vi "Data write draft.vi"() -> ()   [LabVIEW 2012]
uses:
  <vilib>/Platform/TimedLoop/XDataNode/timing_clust.ctl
  <vilib>/Platform/TimedLoop/XDataNode/nitl_modes.ctl
  <vilib>/Platform/TimedLoop/XDataNode/wakeup.ctl
  Labview_Spring2014/EXO200-LabView Dec.8/LabView Dec.8/SubVi's/Connection Variable 1.vi
  <vilib>/addons/database/Connection.llb/Conn Execute.vi
  <vilib>/addons/database/Recordset.llb/Rec Destroy - Connection.vi
  <vilib>/Platform/TimedLoop/XDataNode/XDataNode.xnode
  <vilib>/addons/database/NI_Database_API.lvlib
  Labview_Spring2014/SQL project lib.lvlib
  <vilib>/Platform/TimedLoop/XDataNode/XDNodeRunTimeDep.lvlib
panel:
  out "Time":string
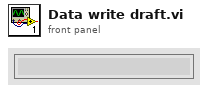
[diagram p1: front panel]
types:
  T1 = typedef "XDNodeRunTimeDep.lvlib/timing_clust.ctl" = cluster{"Expected End [f-1]":u64, "Actual End [f-1]":u64, "Finished Late? [f-1]":bool, "Expected End [i-1]":u64, "Actual End [i-1]":u64, "Finished Late? [i-1]":bool, "Expected Start [i]":u64, "Actual Start [i]":u64, "Expected Start [f]":u64, "Actual Start [f]":u64, "Source Name":string, "Structure Name":string, "Period":i64, "Deadline":i64, "Offset":i64, "Start":i64, "Priority":i32, "Timeout":i32, "Mode":T2, "Wakeup Reason":T3, "Error":errorcluster, "Source Type":string, "Secondary Source Type":string, "Global End Time":u64, "Global Start Time":u64, "Frame Duration":u64, "Iteration Duration":u64, "Assigned CPU":i32, "I/O Scan Engine Mode":u32}
  T2 = typedef "XDNodeRunTimeDep.lvlib/nitl_modes.ctl" = enum32{"No Change", "Process missed periods, maintain original phase", "Discard missed periods, maintain original phase", "Process missed periods, ignore original phase", "Discard missed periods, ignore original phase"}
  T3 = typedef "XDNodeRunTimeDep.lvlib/wakeup.ctl" = enum32{"Normal", "Aborted", "Asynchronous wakeup", "Timing source error", "Timed loop error", "Timeout"}
  T4 = typedef "NI_Database_API.lvlib/Conn ObjectReference.ctl" = refnum<k1>
  T5 = typedef "NI_Database_API.lvlib/Rec ObjectReference.ctl" = refnum<k1>
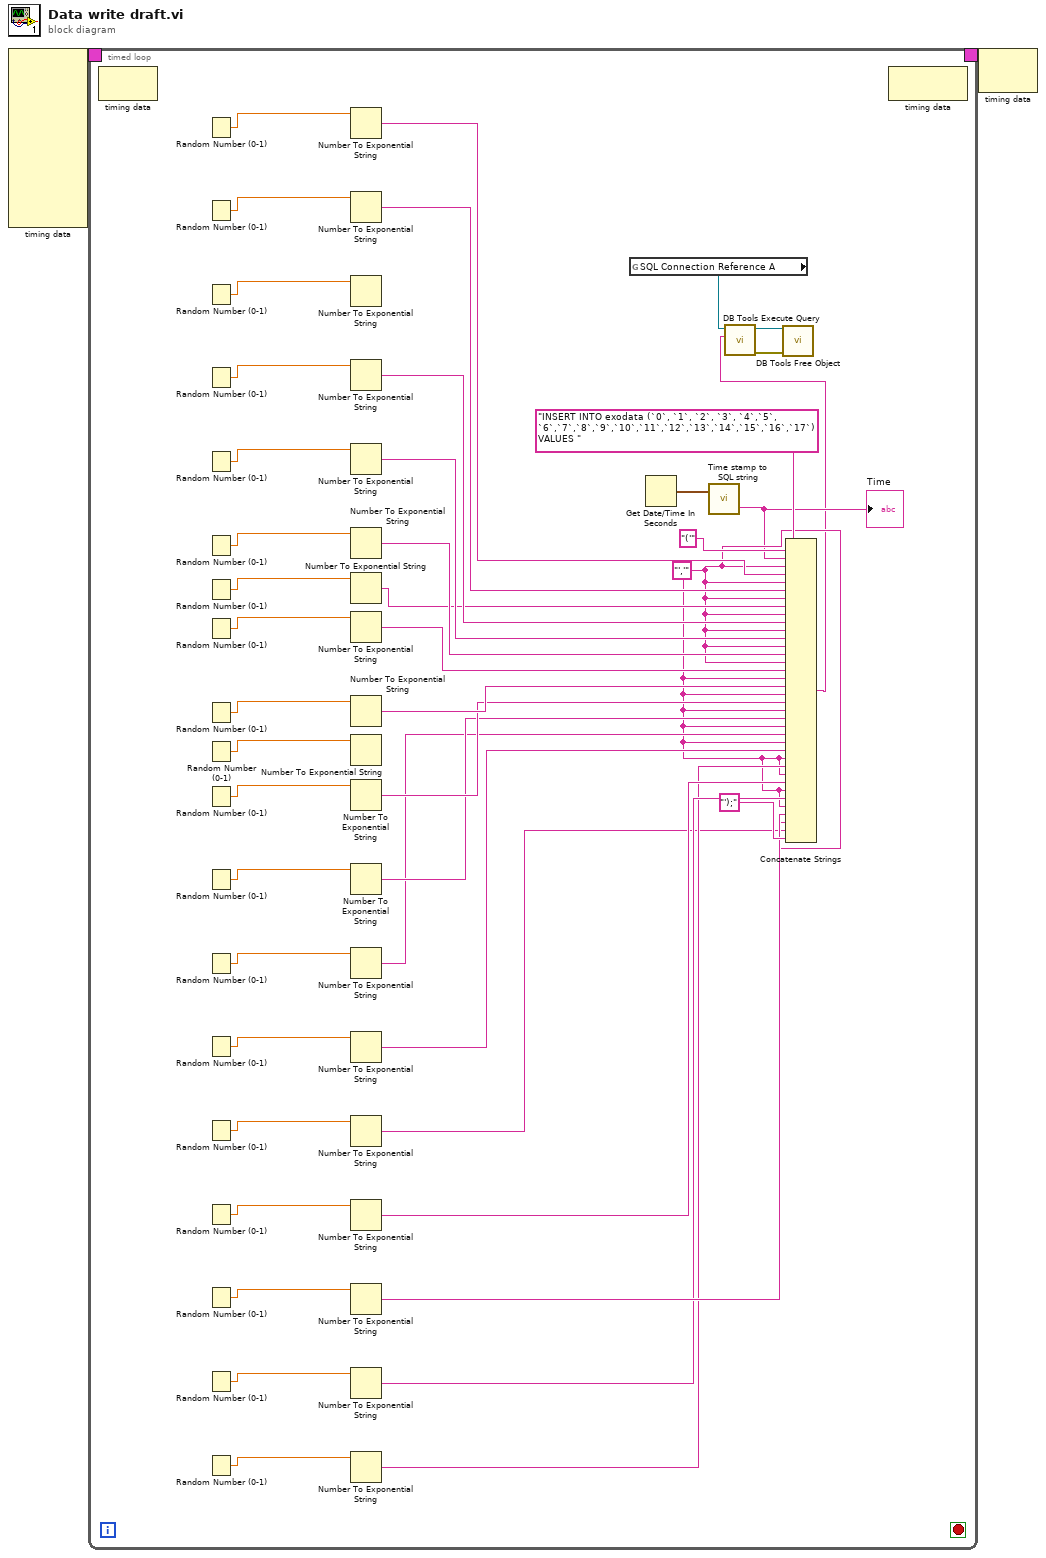
[diagram p0: block diagram]
diagram:
  n1 = node-c288() -> (w2:T1)  [unwired: 10 in]
  n2 = timed-loop {
    timing: w2 -> [_]
    timing-out: [_] -> w1
    stop <- _ stop-if-true
    w5 = "','" ("string")
    n3 = node-c288() -> ()  [unwired: 1 in, 1 out]
    n4 = Random Number (0-1)() -> (number: 0 to 1=w9:dbl)
    n5 = Random Number (0-1)() -> (number: 0 to 1=w10:dbl)
    n6 = Random Number (0-1)() -> (number: 0 to 1=w11:dbl)
    n7 = Random Number (0-1)() -> (number: 0 to 1=w12:dbl)
    n8 = Random Number (0-1)() -> (number: 0 to 1=w13:dbl)
    n9 = Random Number (0-1)() -> (number: 0 to 1=w14:dbl)
    n10 = Random Number (0-1)() -> (number: 0 to 1=w8:dbl)
    n11 = Random Number (0-1)() -> (number: 0 to 1=w15:dbl)
    n12 = Random Number (0-1)() -> (number: 0 to 1=w16:dbl)
    n13 = Random Number (0-1)() -> (number: 0 to 1=w7:dbl)
    n14 = Random Number (0-1)() -> (number: 0 to 1=w17:dbl)
    n15 = Random Number (0-1)() -> (number: 0 to 1=w18:dbl)
    n16 = Random Number (0-1)() -> (number: 0 to 1=w19:dbl)
    n17 = Random Number (0-1)() -> (number: 0 to 1=w20:dbl)
    n18 = Random Number (0-1)() -> (number: 0 to 1=w21:dbl)
    n19 = Random Number (0-1)() -> (number: 0 to 1=w22:dbl)
    n20 = Random Number (0-1)() -> (number: 0 to 1=w23:dbl)
    n21 = Random Number (0-1)() -> (number: 0 to 1=w24:dbl)
    n22 = Random Number (0-1)() -> (number: 0 to 1=w25:dbl)
    n23 = Number To Exponential String(number=w9) -> (E-format string=w42:string)  [unwired: 3 in]
    n24 = Number To Exponential String(number=w10) -> (E-format string=w40:string)  [unwired: 3 in]
    n25 = Number To Exponential String(number=w11) -> ()  [unwired: 3 in, 1 out]
    n26 = Number To Exponential String(number=w12) -> (E-format string=w39:string)  [unwired: 3 in]
    n27 = Number To Exponential String(number=w13) -> (E-format string=w38:string)  [unwired: 3 in]
    n28 = Number To Exponential String(number=w14) -> (E-format string=w37:string)  [unwired: 3 in]
    n29 = Number To Exponential String(number=w8) -> (E-format string=w6:string)  [unwired: 3 in]
    n30 = Number To Exponential String(number=w15) -> (E-format string=w36:string)  [unwired: 3 in]
    n31 = Number To Exponential String(number=w16) -> (E-format string=w35:string)  [unwired: 3 in]
    n32 = Number To Exponential String(number=w7) -> ()  [unwired: 3 in, 1 out]
    n33 = Number To Exponential String(number=w17) -> (E-format string=w34:string)  [unwired: 3 in]
    n34 = Number To Exponential String(number=w18) -> (E-format string=w33:string)  [unwired: 3 in]
    n35 = Number To Exponential String(number=w19) -> (E-format string=w32:string)  [unwired: 3 in]
    n36 = Number To Exponential String(number=w20) -> (E-format string=w31:string)  [unwired: 3 in]
    n37 = Number To Exponential String(number=w21) -> (E-format string=w26:string)  [unwired: 3 in]
    n38 = Number To Exponential String(number=w22) -> (E-format string=w29:string)  [unwired: 3 in]
    n39 = Number To Exponential String(number=w23) -> (E-format string=w30:string)  [unwired: 3 in]
    n40 = Number To Exponential String(number=w24) -> (E-format string=w28:string)  [unwired: 3 in]
    n41 = Number To Exponential String(number=w25) -> (E-format string=w27:string)  [unwired: 3 in]
    n42 = global read "Connection Variable 1.vi" "SQL Connection Reference A"() -> (w44:T4)
    n43 = Get Date/Time In Seconds() -> (seconds since 1Jan1904=w41:timestamp)
    n44 = call "Time stamp to SQL string.vi"("time stamp"=w41) -> ("SQL format date-time string"=w4:string)  [unwired: 1 in, 1 out]
    "Time" <- w4
    n45 = Concatenate Strings("INSERT INTO exodata (`0`, `1`, `2`, `3`, `4`,`5`, `6`,`7`,`8`,`9`,`10`,`11`,`12`,`13`,`14`,`15`,`16`,`17`) VALUES ", "('" ("string"), w4, w5, w42, w5, w40, w5, w6, w5, w39, w5, w38, w5, w37, w5, w36, w5, w35, w5, w34, w5, w33, w5, w32, w5, w31, w5, w27, w5, w29, w5, w28, w5, w30, w5, w26, "');" ("string")) -> (w3:string)
    n46 = call-poly <vilib>:"DB Tools Execute Query.vi"("SQL query"=w3, "connection reference"=w44) -> ("error out"=w43:errorcluster, "recordset reference"=w45:T5)  [unwired: 6 in]
    n47 = call-poly <vilib>:"DB Tools Free Object.vi"("error in (no error)"=w43, "recordset reference"=w45) -> ()  [unwired: 10 out]
    n48 = node-c288() -> ()  [unwired: 1 in, 1 out]
  }
  n49 = node-c288(w1) -> ()  [unwired: 1 out]
